vi "AutoShooter.vi"(0 "Clapper":T1={"DevStatus"={"status"=FALSE, "code"=0, "source"=""}, "Solenoid Module"=enum."Solenoid Module 1", "Forward Solenoid Channel"=enum."Invalid", "Reverse Solenoid Channel"=enum."Invalid"}, 1 "Roller":T1={"DevStatus"={"status"=FALSE, "code"=0, "source"=""}, "Solenoid Module"=enum."Solenoid Module 1", "Forward Solenoid Channel"=enum."Invalid", "Reverse Solenoid Channel"=enum."Invalid"}, 2 "Kicker":T1={"DevStatus"={"status"=FALSE, "code"=0, "source"=""}, "Solenoid Module"=enum."Solenoid Module 1", "Forward Solenoid Channel"=enum."Invalid", "Reverse Solenoid Channel"=enum."Invalid"}, 3 "FiringCylinder":T1={"DevStatus"={"status"=FALSE, "code"=0, "source"=""}, "Solenoid Module"=enum."Solenoid Module 1", "Forward Solenoid Channel"=enum."Invalid", "Reverse Solenoid Channel"=enum."Invalid"}, 5 "error in":errorcluster, 6 "Action":T4, 7 "Wait1":u32, 9 "Wait2":u32, 11 "Wait3":u32, 13 "CheckCollectorArm?":bool=TRUE) -> (19 "error out":errorcluster)   [LabVIEW 2013]
doc: "AutoShooter has the following actions:\n-Init: take two double solenoid references and store them (one for the clapper, one for the roller). Take two single solenoid references and use them to initialize Shooter.vi (one for the firing cylinder, one for the kicker).\n-Shoot:\n +Check if the collector is up (hitting the top limit switch). (Only if CheckLimitSwitch is true.)\n +Actuate the roller to out.\n +Actuate the clapper to middle.\n +Shoot (using Shooter.vi). Wait1, Wait2, and Wait3 correspond to the waits used by Shooter.vi."
uses:
  ShooterAction.ctl
  AutoShooterAction.ctl
  <vilib>/Rock Robotics/WPI/Solenoid/WPI_SolenoidChannel.ctl
  <vilib>/Rock Robotics/SystemInterfaces/Typedef/FPGA_TypedefSolenoidModule.ctl
  <vilib>/Rock Robotics/WPI/Solenoid/WPI_SolenoidDevRef.ctl
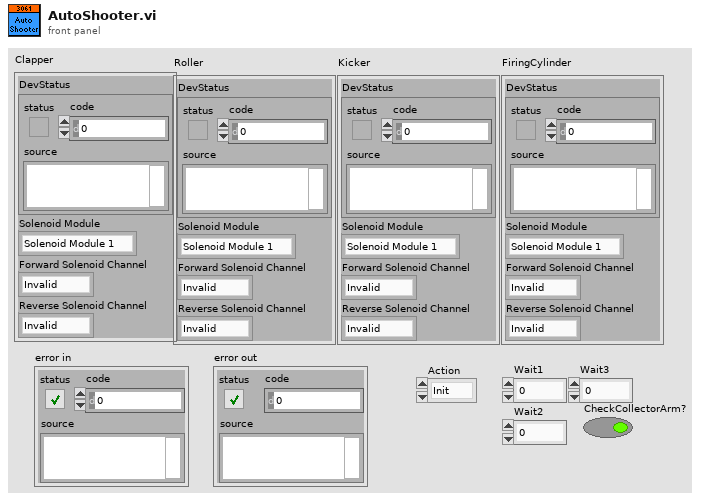
[diagram p1: front panel]
types:
  T1 = typedef "WPI_SolenoidDevRef.ctl" = cluster{"DevStatus":errorcluster, "Solenoid Module":T2, "Forward Solenoid Channel":T3, "Reverse Solenoid Channel":T3}
  T2 = typedef "FPGA_TypedefSolenoidModule.ctl" = enum16{"Solenoid Module 1", "Solenoid Module 2"}
  T3 = typedef "WPI_SolenoidChannel.ctl" = enum8{"Solenoid 1", "Solenoid 2", "Solenoid 3", "Solenoid 4", "Solenoid 5", "Solenoid 6", "Solenoid 7", "Solenoid 8", "Invalid"}
  T4 = typedef "AutoShooterAction.ctl" = enum16{"Init", "Shoot"}
  T5 = typedef "ShooterAction.ctl" = enum16{"Init", "Shoot"}
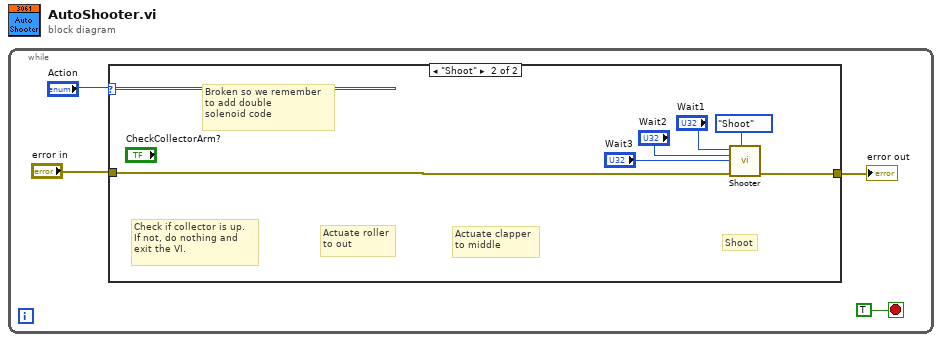
[diagram p0: block diagram]
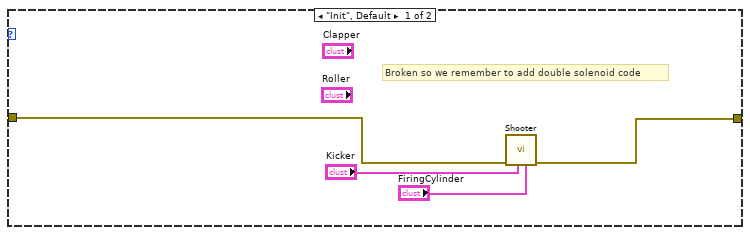
[diagram p2: hidden frame]
diagram:
  n1 = while {
    stop <- TRUE stop-if-true
    n2 = case shown="\"Shoot\"" "Action" {
      tunnel: "error in" -> [w6 w11]
      tunnel: [w5 w16] -> w1
      frame "Init", Default {
        # "Broken so we remember to add double solenoid code"
        n3 = call "Shooter.vi"("FiringCylinder"="FiringCylinder", "Kicker"="Kicker", "error in"=w6) -> ("error out"=w5:errorcluster)  [unwired: 8 in]
      }
      frame "Shoot" {
        # "Broken so we remember\nto add double\nsolenoid code"
        # "Shoot"
        # "Actuate clapper\nto middle"
        # "Actuate roller\nto out"
        # "Check if collector is up.\nIf not, do nothing and\nexit the VI."
        n4 = call "Shooter.vi"("Action"=ShooterAction."Shoot", "error in"=w11, "Wait3"="Wait3", "Wait2"="Wait2", "Wait1"="Wait1") -> ("error out"=w16:errorcluster)  [unwired: 6 in]
      }
    }
    "error out" <- w1
  }
